vi "Start Inspect 2.vi"(6 "wait for reply (T)":bool=TRUE, 8 "error in (no error)":errorcluster, 10 "Start(T)/Stop(F)":bool) -> (0 "error out":errorcluster, 1 "timed out?":bool, 2 "Reply Payload":T1)   [LabVIEW 2015, in "Tool Module.lvlib"]
doc: "Starts a new inspection cycle. The request replies with a reference to the sample data notifier, which includes status bits and sample data. The notifier is updated as the tool moves and collects data.\n_____\nCreated using Delacor QMH Event Scripter 4.2.1.88."
uses:
  Tool Module.lvlib
  Start Inspect 2 (Reply Payload)--cluster.ctl
  Support/_Sample Data Rtn Cluster--typedef.ctl
  Start Inspect 2 Argument--cluster.ctl
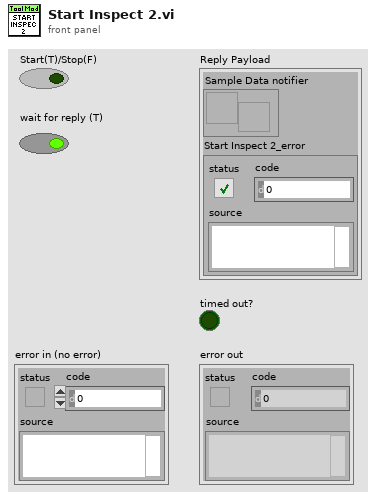
[diagram p1: front panel]
types:
  T1 = typedef "Tool Module.lvlib/Start Inspect 2 (Reply Payload)--cluster.ctl" = cluster{"Sample Data notifier":refnum<notifier>, "Start Inspect 2_error":errorcluster}
  T2 = typedef "Tool Module.lvlib/Start Inspect 2 Argument--cluster.ctl" = cluster{"Start(T)/Stop(F)":bool, "Wait Notifier":refnum<notifier>, "wait for reply":bool}
  T3 = typedef "Tool Module.lvlib/Request Events--cluster.ctl" = cluster{"Stop Module":refnum<user-event>, "Show Panel":refnum<user-event>, "Hide Panel":refnum<user-event>, "Get Module Execution Status":refnum<user-event>, "Show Diagram":refnum<user-event>, "GOTO":refnum<user-event>, "Start Inspect":refnum<user-event>, "CONNECT":refnum<user-event>, "Get All Inspect Data":refnum<user-event>, "Start Data Monitor":refnum<user-event>, "Get FPGA Setup Params":refnum<user-event>, "Set FPGA Setup Params":refnum<user-event>, "Commit Tool Config":refnum<user-event>, "Set Integration Count":refnum<user-event>, "Set Laser Params":refnum<user-event>, "Get Mtrl Ctrl Reg":refnum<user-event>, "Commit Ctrl Reg":refnum<user-event>, "Set Event Logger":refnum<user-event>, "Write to File":refnum<user-event>, "Read from File":refnum<user-event>, "Set Device Temp Thresholds":refnum<user-event>, "Get Cycle Count":refnum<user-event>, "Return FPGA Setup Data":refnum<user-event>, "Update FPGA Setup Data":refnum<user-event>, "Setup Timer":refnum<user-event>, "Tool Status Reader Cmd":refnum<user-event>, "Stop Helper Loops":refnum<user-event>, "Enable Receive Stream":refnum<user-event>, "Get-Set Inspection Limits":refnum<user-event>, "Start Inspect 2":refnum<user-event>}
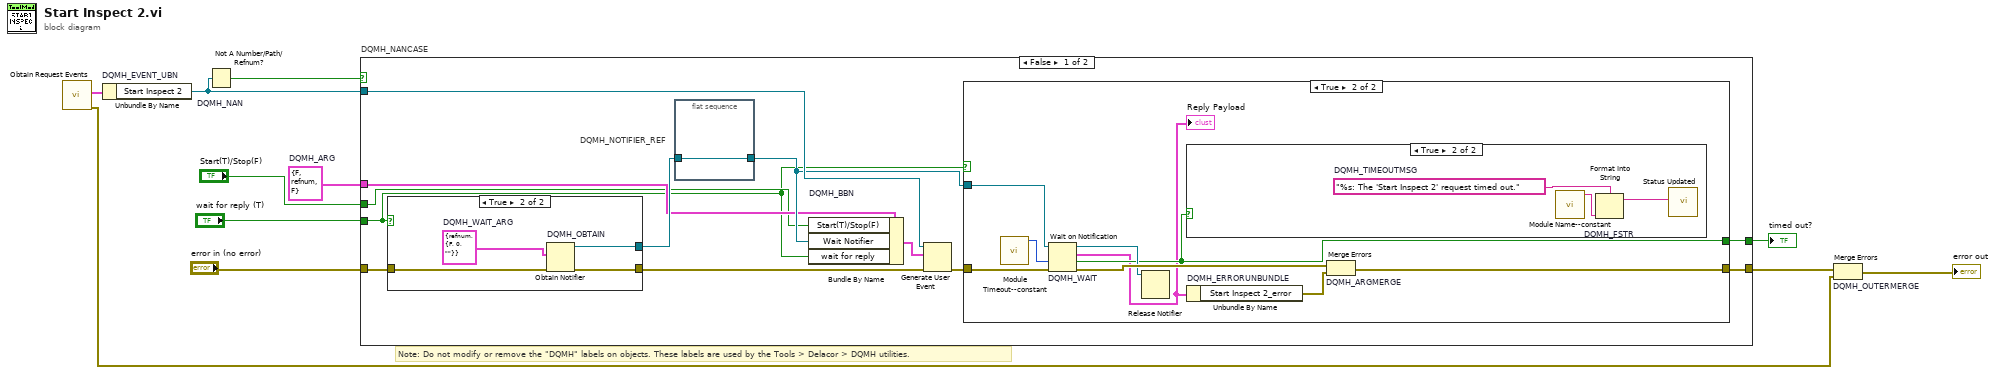
[diagram p0: block diagram]
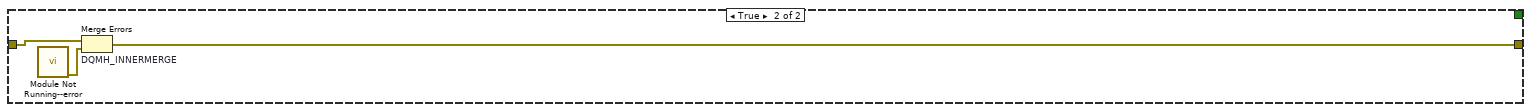
[diagram p5: hidden frame]
diagram:
  w5 = T2 {"Start(T)/Stop(F)"=FALSE, "Wait Notifier"=refnum, "wait for reply"=FALSE}  # DQMH_ARG
  # "Note: Do not modify or remove the \"DQMH\" labels on objects. These labels are used by the Tools > Delacor > DQMH utilities."
  n1 = call "Obtain Request Events.vi"() -> ("error out"=w2:errorcluster, "Tool Module Request Events"=w1:T3)  [unwired: 10 in]
  n2 = Unbundle By Name "DQMH_EVENT_UBN"(w1) -> ("Start Inspect 2"=w9:refnum<user-event>)
  n3 = Not A Number/Path/Refnum? "DQMH_NAN"(number/path/refnum=w9) -> (NaN/Path/Refnum?=w8:bool)
  n4 = case "DQMH_NANCASE" shown="False" w8 {
    tunnel: "error in (no error)" -> [w23 w45]
    tunnel: w9 -> [w21 _]
    tunnel: [w18 w44] -> w6
    tunnel: [w19 _] -> w7
    tunnel: w5 -> [w14 _]
    tunnel: "Start(T)/Stop(F)" -> [w13 _]
    tunnel: "wait for reply (T)" -> [w12 _]
    frame False {
      n5 = case shown="True" w12 {
        tunnel: w23 -> [w38 w42]
        tunnel: [w38 w41] -> w20
        tunnel: [_ w39] -> w16
        frame False {
        }
        frame True {
          w40 = T1 {"Sample Data notifier"=refnum, "Start Inspect 2_error"={"status"=FALSE, "code"=0, "source"=""}}  # DQMH_WAIT_ARG
          n6 = Obtain Notifier "DQMH_OBTAIN"(notification data type=w40, error in (no error)=w42) -> (notifier out=w39:refnum<notifier>, error out=w41:errorcluster)  [unwired: 2 in, 1 out]
        }
      }
      n7 = flat-sequence "DQMH_NOTIFIER_REF" {
        tunnel: w16 -> [w24]
        tunnel: [w24] -> w15
        frame #0 {
        }
      }
      n8 = Bundle By Name "DQMH_BBN"(cluster=w14, "Start(T)/Stop(F)"=w13, "Wait Notifier"=w15, "wait for reply"=w12) -> (w17:T2)
      n9 = Generate User Event(user event=w21, event data cluster=w17, error in=w20) -> (error out=w22:errorcluster)  [unwired: 1 in, 1 out]
      n10 = case shown="True" w12 {
        tunnel: w22 -> [w25 w34]
        tunnel: w15 -> [_ w32]
        tunnel: [_ w30] -> w19
        tunnel: [w25 w29] -> w18
        frame False {
        }
        frame True {
          n11 = call "Module Timeout--constant.vi"() -> ("Module Timeout"=w26:i32)  [unwired: 11 in]
          n12 = Wait on Notification "DQMH_WAIT"(notifier=w32, timeout in ms (-1)=w26, error in (no error)=w34) -> (notifier out=w31:refnum<notifier>, notification=w27:T1, timed out?=w30:bool, error out=w33:errorcluster)  [unwired: 1 in]
          "Reply Payload" <- w27
          n13 = Release Notifier(notifier=w31) -> ()  [unwired: 2 in, 3 out]
          n14 = case shown="True" w30 {
            frame False {
            }
            frame True {
              w37 = "%s: The 'Start Inspect 2' request timed out."  # DQMH_TIMEOUTMSG
              n15 = call "Module Name--constant.vi"() -> ("Module Name"=w36:string)  [unwired: 11 in]
              n16 = Format Into String "DQMH_FSTR"(format string=w37, w36) -> (resulting string=w35:string)  [unwired: 2 in, 1 out]
              n17 = call "Status Updated.vi"("Status"=w35) -> ()  [unwired: 10 in, 1 out]
            }
          }
          n18 = Unbundle By Name "DQMH_ERRORUNBUNDLE"(w27) -> ("Start Inspect 2_error"=w28:errorcluster)
          n19 = Merge Errors "DQMH_ARGMERGE"(w33, w28) -> (w29:errorcluster)
        }
      }
    }
    frame True {
      n20 = call "Module Not Running--error.vi"() -> ("error out"=w43:errorcluster)  [unwired: 11 in]
      n21 = Merge Errors "DQMH_INNERMERGE"(w45, w43) -> (w44:errorcluster)
    }
  }
  "timed out?" <- w7
  n22 = Merge Errors "DQMH_OUTERMERGE"(w6, w2) -> (→"error out":errorcluster)
